vi "Verify Hello World.vi"(8 "error in":errorcluster) -> (0 "error out":errorcluster)   [LabVIEW 2020, in "Caraya Extension Tests.lvclass"]
uses:
  Caraya Extension Tests.lvclass
  Source/Approval Tests/Options/Options.lvclass/Options.ctl
  Source/Approval Tests/Naming Data/Naming Data.lvclass/Naming Data.ctl
  4b862e9e-fcb2-487f-ab73-d9f83fbf4d2c.vi
  4b862e9e-fcb2-487f-ab73-d9f83fbf4d2c.vi/500b534b-d6f0-4fa5-90b2-c40158375321.vi
  Source/Approval Tests/Replace if Empty.vi
  Source/Approval Tests/Options/Update Test Name if Not Defined.vi
  Source/Approval Tests/Verify Core.vi
  4b862e9e-fcb2-487f-ab73-d9f83fbf4d2c.vi/500b534b-d6f0-4fa5-90b2-c40158375321.vi/93c5622b-9fb7-41e0-8c76-3fde37e94e34.vi
  Source/Approval Tests/Options/Read Scrubber.vi
  Source/Approval Tests/Naming Data/Read Test VI Name.vi
  Source/Approval Tests/Naming Data/Write Test VI Name.vi
  Source/Approval Tests/Options/Read Namer.vi
  Source/Approval Tests/Options/Read Naming Data.vi
  Source/Approval Tests/Options/Read Reporter.vi
  Source/Approval Tests/Options/Read Text Comparator.vi
  4b862e9e-fcb2-487f-ab73-d9f83fbf4d2c.vi/500b534b-d6f0-4fa5-90b2-c40158375321.vi/93c5622b-9fb7-41e0-8c76-3fde37e94e34.vi/04cb982b-2eda-40d0-8d7e-90f8e0b569b2.vi
  Source/Approval Tests/Options/Add Label to Namer.vi
  Source/Approval Tests/conv EOL.vi
  <vilib>/Utility/libraryn.llb/Check if File or Folder Exists.vi
  Source/Approval Tests/Reporter/Report.vi
  <vilib>/addons/_JKI Toolkits/Caraya/classes/Assert/Assert.vi
  <vilib>/addons/_JKI Toolkits/Caraya/classes/Assert/Assert True.vi
  Source/Approval Tests/Scrubber/Scrubber.lvclass
  Source/Approval Tests/Namer/Namer.lvclass
  Source/Approval Tests/Naming Data/Naming Data.lvclass
  Source/Approval Tests/Reporter/Reporter.lvclass
  Source/Approval Tests/Text Comparator/Text Comparator.lvclass
  Source/Approval Tests/Options/Options.lvclass
  <vilib>/addons/_JKI Toolkits/Caraya/classes/Test/Test.lvclass
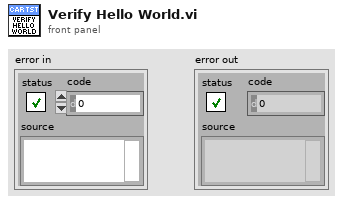
[diagram p1: front panel]
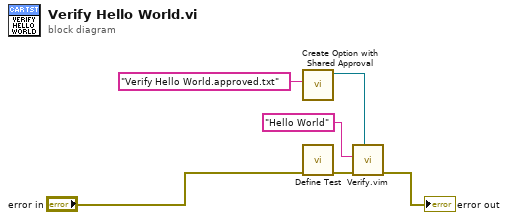
[diagram p0: block diagram]
diagram:
  n1 = call "Create Option with Shared Approval.vi"("Filename"="Verify Hello World.approved.txt") -> ("Options outs"=w1:refnum<class "Options.lvclass">)  [unwired: 10 in]
  n2 = call <vilib>:"Define Test.vi"("error in (no error)"="error in") -> ("error out"=w6:errorcluster)  [unwired: 9 in, 1 out]
  n3 = call "Verify.vim"("Options"=w1, "error in"=w6, "Test Data"="Hello World") -> ("error out"=→"error out":errorcluster)  [unwired: 7 in, 1 out]
